vi "verifyMotorController.vi"(8 "error in (no error)":errorcluster, 10 "interface object in":refnum<k20>, 11 "MotorController in":refnum<class "MotorController.lvclass">) -> (0 "error out":errorcluster, 1 "isCorrectController":bool, 2 "interface object out":refnum<k20>, 3 "MotorController out":refnum<class "MotorController.lvclass">)   [LabVIEW 2018, in "MotorController.lvclass"]
uses:
  MotorController.lvclass
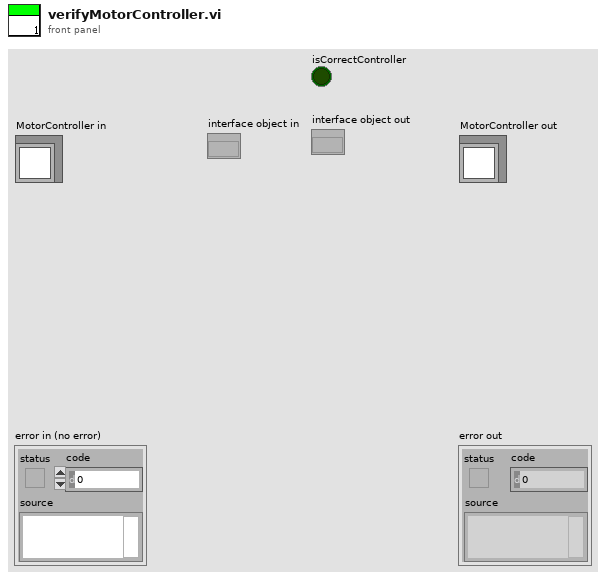
[diagram p1: front panel]
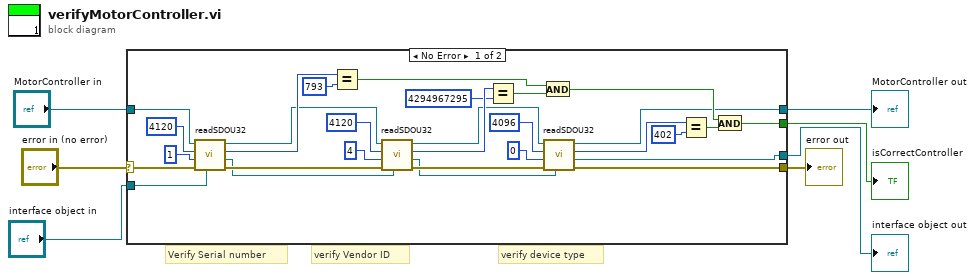
[diagram p0: block diagram]
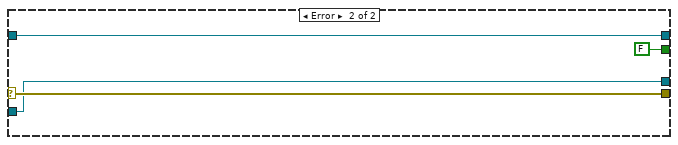
[diagram p2: hidden frame]
diagram:
  # "verify device type"
  # "Verify Serial number"
  # "verify Vendor ID"
  n1 = case shown="No Error" "error in (no error)" {
    selector: "error in (no error)" -> [w35 w40]
    tunnel: [w8 w40] -> w6
    tunnel: [w9 w39] -> w4
    tunnel: "MotorController in" -> [w34 w39]
    tunnel: [w10 w37] -> w3
    tunnel: "interface object in" -> [w36 w37]
    tunnel: [w15 FALSE] -> w1
    frame No Error {
      n2 = call "readSDOU32.vi"("interface object in"=w36, "error in (no error)"=w35, "subIndex"=u8 1, "objectIndex"=u16 4120, "MotorController in"=w34) -> ("error out"=w22:errorcluster, "interface object out"=w21:refnum<k20>, "output"=w31:u32, "MotorController out"=w25:refnum<class "MotorController.lvclass">)  [unwired: 3 in]
      n3 = Equal?(x=w31, y=u32 793) -> (x = y?=w29:bool)
      n4 = call "readSDOU32.vi"("interface object in"=w21, "error in (no error)"=w22, "subIndex"=u8 4, "objectIndex"=u16 4120, "MotorController in"=w25) -> ("error out"=w17:errorcluster, "interface object out"=w11:refnum<k20>, "output"=w27:u32, "MotorController out"=w20:refnum<class "MotorController.lvclass">)  [unwired: 3 in]
      n5 = Equal?(x=w27, y=u32 4294967295) -> (x = y?=w28:bool)
      n6 = And(x=w29, y=w28) -> (x .and. y?=w16:bool)
      n7 = call "readSDOU32.vi"("interface object in"=w11, "error in (no error)"=w17, "subIndex"=u8 0, "objectIndex"=u16 4096, "MotorController in"=w20) -> ("error out"=w8:errorcluster, "interface object out"=w10:refnum<k20>, "output"=w14:u32, "MotorController out"=w9:refnum<class "MotorController.lvclass">)  [unwired: 3 in]
      n8 = Equal?(x=w14, y=u32 402) -> (x = y?=w12:bool)
      n9 = And(x=w16, y=w12) -> (x .and. y?=w15:bool)
    }
    frame Error {
    }
  }
  "error out" <- w6
  "MotorController out" <- w4
  "interface object out" <- w3
  "isCorrectController" <- w1
